vi "ex7_softtrig_model_b.vi"() -> ()   [LabVIEW 2012]
uses:
  <userlib>/QI_Transition.llb/QCam Grab Abort.vi
panel:
  in  "Trigger":bool
  in  "Halt loop":bool
  in  "stop":bool
  out "error status":errorcluster
  out "Preview Window":picture
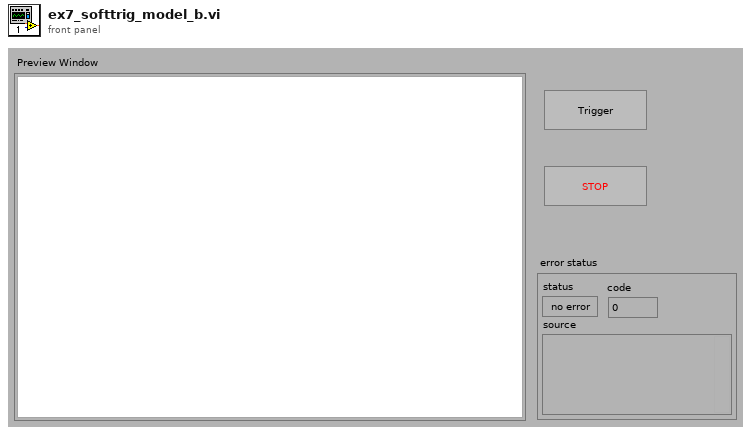
[diagram p1: front panel]
types:
  T1 = enum32{"Freerun", "Edge hi", "Edge low", "Pulse hi", "Pulse low", "Software"}
  T2 = typedef "IMAQ Image.ctl" = refnum<image>
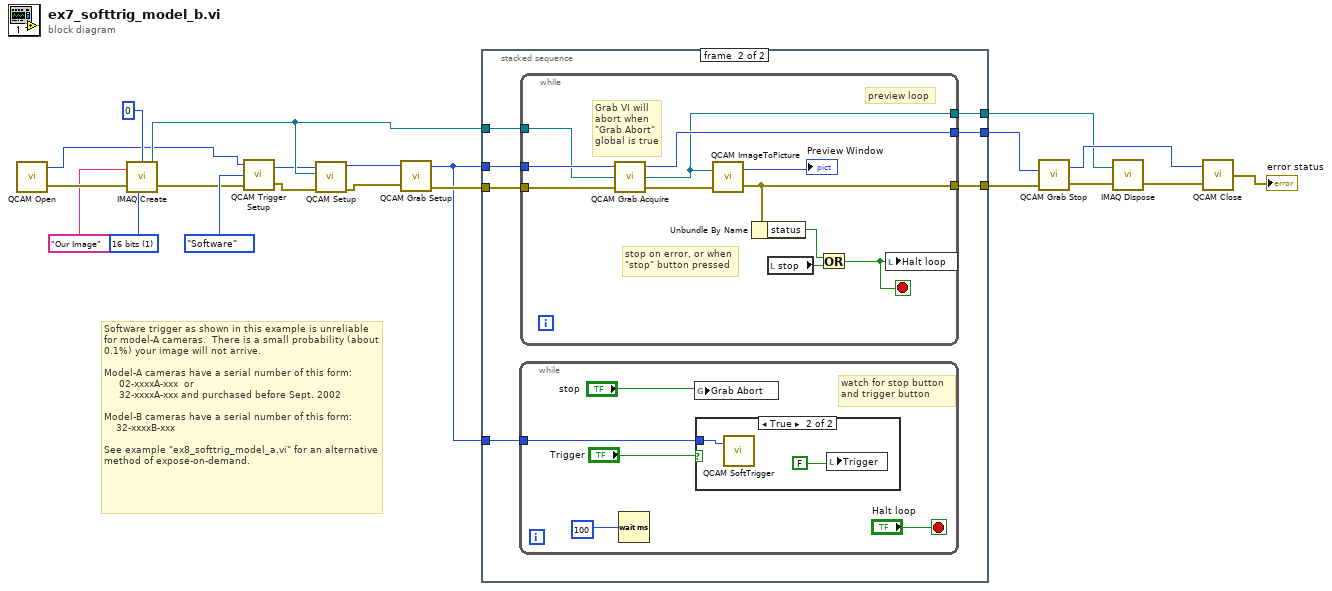
[diagram p0: block diagram]
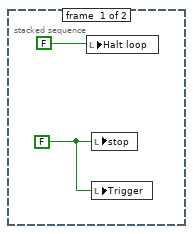
[diagram p2: hidden frame]
diagram:
  w7 = u32 1 items=["8 bits", "16 bits"] ("Image Type")
  # "Software trigger as shown in this example is unreliable for model-A cameras.  There is a small probability (about 0.1%) your image will not arrive.\n\nModel-A cameras have a serial number of this form:\n     02-xxxxA-xxx  or \n     32-xxxxA-xxx and purchased before Sept. 2002  \n\nModel-B cameras have a serial number of this form:\n    32-xxxxB-xxx\n\nSee example \"ex8_softtrig_model_a.vi\" for an alternative method of expose-on-demand."
  n1 = call <userlib>:"QCAM Open.vi"() -> ("error out"=w21:errorcluster, "cameraId out"=w1:u32)  [unwired: 2 in]
  n2 = call "IMAQ Create"("Border Size"=0, "Image Name"="Our Image", "Image Type"=w7, "error in (no error)"=w21) -> ("New Image"=w16:T2, "error out"=w6:errorcluster)  [unwired: 1 out]
  n3 = call <userlib>:"QCAM Trigger Setup.vi"("error in (no error)"=w6, "trigger mode"=T1."Software" ("Trigger Mode"), "camera Id"=w1) -> ("error out"=w5:errorcluster, "camera Id out"=w4:u32)
  n4 = call <userlib>:"QCAM Setup.vi"("error in (no error)"=w5, "Image"=w16, "cameraId"=w4) -> ("error out"=w2:errorcluster, "cameraId out"=w3:u32)  [unwired: 3 in, 4 out]
  n5 = call <userlib>:"QCAM Grab Setup.vi"("error in (no error)"=w2, "cameraId"=w3) -> ("error out"=w17:errorcluster, "cameraId out"=w9:u32)
  n6 = stacked-sequence {
    tunnel: w17 -> [_ w30]
    tunnel: w9 -> [_ w29]
    tunnel: w16 -> [_ w28]
    tunnel: [_ w27] -> w15
    tunnel: [_ w26] -> w14
    tunnel: [_ w25] -> w11
    tunnel: w9 -> [_ w24]
    frame #0 {
      w22 = FALSE
      n7 = local write "Halt loop"(FALSE) -> ()
      n8 = local write "stop"(w22) -> ()
      n9 = local write "Trigger"(w22) -> ()
    }
    frame #1 {
      n10 = while {
        tunnel: w24 -> [w43]
        stop <- "Halt loop" stop-if-true
        # "watch for stop button\nand trigger button"
        n11 = Wait (ms)(milliseconds to wait=100) -> ()  [unwired: 1 out]
        n12 = global write "QCam Grab Abort.vi" "Grab Abort"("stop") -> ()
        n13 = case shown="True" "Trigger" {
          tunnel: w43 -> [_ w47]
          frame False {
          }
          frame True {
            n14 = call <userlib>:"QCAM SoftTrigger.vi"("cameraId"=w47) -> ()  [unwired: 1 in, 2 out]
            n15 = local write "Trigger"(FALSE) -> ()
          }
        }
      }
      n16 = while {
        tunnel: [w36] -> w25
        tunnel: [w33] -> w27
        tunnel: w28 -> [w34]
        tunnel: w29 -> [w35]
        tunnel: w30 -> [w38]
        tunnel: [w39] -> w26
        stop <- w31 stop-if-true
        # "Grab VI will abort when \"Grab Abort\" global is true"
        # "preview loop"
        # "stop on error, or when \"stop\" button pressed"
        n17 = call <userlib>:"QCAM Grab Acquire.vi"("error in (no error)"=w38, "Image"=w34, "cameraId"=w35) -> ("error out"=w40:errorcluster, "Image Out"=w36:T2, "cameraId out"=w39:u32)
        n18 = call <userlib>:"QCAM ImageToPicture.vi"("error in (no error)"=w40, "Image"=w36) -> ("error out"=w33:errorcluster, "Picture Out"=→"Preview Window":picture)
        n19 = Unbundle By Name(w33) -> ("status"=w37:bool)
        n20 = local read "stop"() -> (w32:bool)
        n21 = Or(x=w37, y=w32) -> (x .or. y?=w31:bool)
        n22 = local write "Halt loop"(w31) -> ()
      }
    }
  }
  n23 = call <userlib>:"QCAM Grab Stop.vi"("error in (no error)"=w15, "cameraId"=w14) -> ("error out"=w20:errorcluster, "cameraId Out"=w18:u32)
  n24 = call "IMAQ Dispose"("Image"=w11, "error in (no error)"=w20) -> ("error out"=w19:errorcluster)  [unwired: 1 in, 3 out]
  n25 = call <userlib>:"QCAM Close.vi"("error in (no error)"=w19, "cameraId"=w18) -> ("error out"=→"error status":errorcluster)
